vi "Polymorphic Children Data.vi"(8 "Error In":errorcluster, 11 "Instance VIs":T1(array[cluster])) -> (0 "Error Out":errorcluster, 3 "Children":refnum<class "Array.lvclass">)   [LabVIEW 2018, in "Scripts.lvlib"]
uses:
  Scripts.lvlib
  Toolkit/Data/Array/Array.lvclass
  D:/Users/cfield/Code/Field R&D Services/Mustache/LabVIEW/trunk/src/Toolkit/Data/Datum/Datum.lvclass
  Toolkit/Data/Map/Map.lvclass
  Toolkit/Data/Pair/Support/From String.vi
  Toolkit/Data/Pair/Support/From Datum.vi
  Toolkit/Data/Map/Support/From Pair Array.vi
  Toolkit/Data/Array/Support/From Data.vi
  Toolkit/Data/Pair/Pair.lvclass
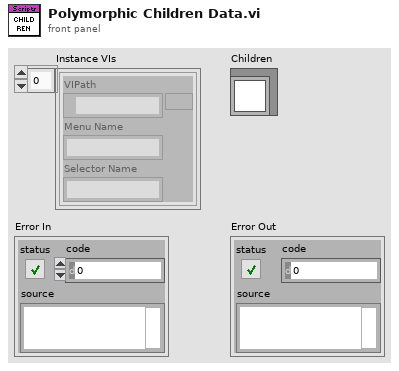
[diagram p1: front panel]
types:
  T1 = cluster{"VIPath":path, "Menu Name":string, "Selector Name":string}[]
  T2 = cluster{"Alt":string, "Description":string, "Src":string}[]
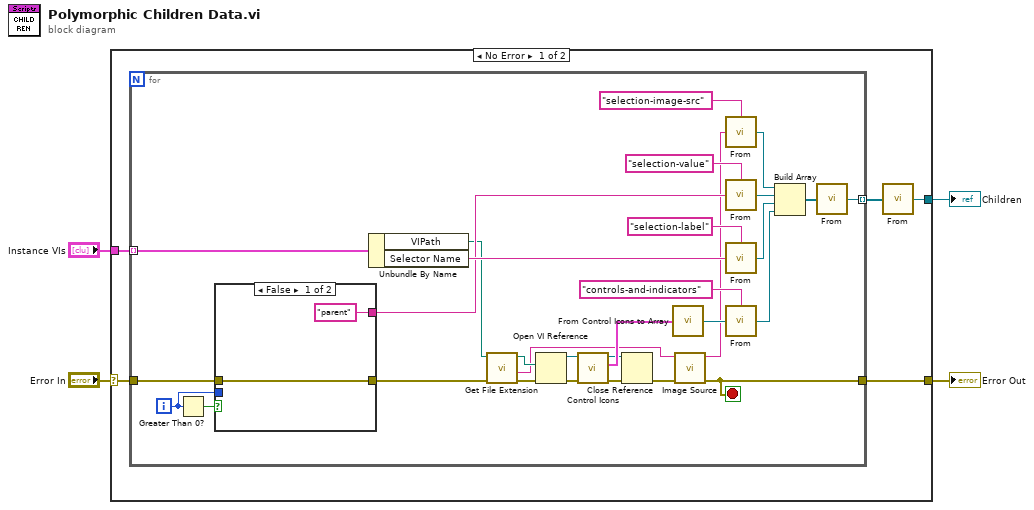
[diagram p0: block diagram]
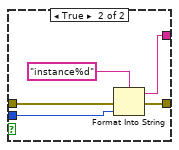
[diagram p2: hidden frame]
diagram:
  n1 = case shown="No Error" "Error In" {
    selector: "Error In" -> [w6 w47]
    tunnel: [w9 _] -> w4
    tunnel: [w5 w47] -> w3
    tunnel: "Instance VIs" -> [w7 _]
    frame No Error {
      n2 = for {
        tunnel: w7 -> [w39] mode=indexing
        tunnel: w6 -> [w24]
        tunnel: [w27] -> w8 mode=indexing
        tunnel: [w12] -> w5
        i -> [w23]
        stop <- w12 stop-if-true
        n3 = Greater Than 0?(x=w23) -> (x > 0?=w25:bool)
        n4 = case shown="False" w25 {
          tunnel: w24 -> [w41 w46]
          tunnel: [w41 w45] -> w17
          tunnel: w23 -> [_ w43]
          tunnel: ["parent" w42] -> w22
          frame False {
          }
          frame True {
            n5 = Format Into String(format string="instance%d", error in=w46, w43) -> (resulting string=w42:string, error out=w45:errorcluster)  [unwired: 1 in]
          }
        }
        n6 = Unbundle By Name(w39) -> ("VIPath"=w19:path, "Selector Name"=w32:string)
        n7 = call <vilib>:"Get File Extension.vi"("error in (no error)"=w17, "file"=w19) -> ("error out"=w16:errorcluster, "filename without extension"=w15:string, "dup file"=w18:path)  [unwired: 5 in, 2 out]
        n8 = Open VI Reference(vi path=w18, error in (no error)=w16) -> (vi reference=w37:refnum<vi>, error out=w38:errorcluster)  [unwired: 4 in]
        n9 = call "Control Icons.vi"("Error In"=w38, "VI In"=w37) -> ("Error Out"=w10:errorcluster, "Control Icons"=w35:T2, "VI Out"=w11:refnum<vi>)  [unwired: 7 in]
        n10 = Close Reference(reference=w11, error in (no error)=w10) -> (error out=w14:errorcluster)
        n11 = call "From Control Icons to Array.vi"("Control Icons"=w35) -> ("Array"=w36:refnum<class "Array.lvclass">)
        n12 = call "Image Source.vi"("Error In"=w14, "Spaced File Stem"=w15) -> ("Error Out"=w12:errorcluster, "Image Src"=w13:string)  [unwired: 8 in]
        n13 = call-poly "From.vi"("Value"=w13, "Key"="selection-image-src") -> ("Pair"=w20:refnum<class "Pair.lvclass">)
        n14 = call-poly "From.vi"("Value"=w22, "Key"="selection-value") -> ("Pair"=w30:refnum<class "Pair.lvclass">)
        n15 = call-poly "From.vi"("Value"=w32, "Key"="selection-label") -> ("Pair"=w29:refnum<class "Pair.lvclass">)
        n16 = call-poly "From.vi"("Value"=w36, "Key"="controls-and-indicators") -> ("Pair"=w28:refnum<class "Pair.lvclass">)
        n17 = Build Array(w20, w30, w29, w28) -> (w26:refnum<class "Pair.lvclass">[])
        n18 = call-poly "From.vi"("Pairs"=w26) -> ("Map"=w27:refnum<class "Map.lvclass">)  [unwired: 1 in]
      }
      n19 = call-poly "From.vi"("Data"=w8) -> ("Array"=w9:refnum<class "Array.lvclass">)  [unwired: 1 in]
    }
    frame Error {
    }
  }
  "Children" <- w4
  "Error Out" <- w3
